vi "Wrapper_setBoxcarWidth.vi"(1 "Boxcar Width":i32, 2 "Index":i32, 3 "Wrapper In":u32) -> (0 "Wrapper Out":u32)   [LabVIEW 2017]
uses:
  OmniDriver32.dll
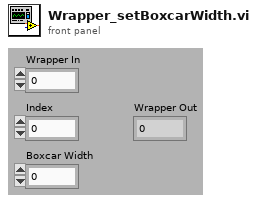
[diagram p1: front panel]
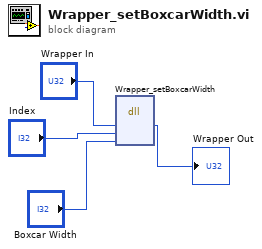
[diagram p0: block diagram]
diagram:
  n1 = dll-call lib="OmniDriver32.dll" fn="Wrapper_setBoxcarWidth" label="Wrapper.setBoxcarWidth"("Wrapper"="Wrapper In", "Index"="Index", "Boxcar Width"="Boxcar Width") -> ("Wrapper"=→"Wrapper Out":u32)  [unwired: 5 in, 3 out]
